vi "CS-4 Status.vi"(0 "VISA session":refnum<visa-resource-name>, 11 "error in (no error)":errorcluster) -> (1 "Magnet Current":string=" +000.000 A                ", 2 "Magnet Voltage":string=" +0.00 V                ", 3 "Output Current":string=" +000.000 A                ", 4 "dup VISA session":refnum<visa-resource-name>, 6 "Output Voltage":string=" +0.00 V                ", 8 "Sweep Mode":string="PAUSED", 9 "sweep states":T1, 10 "Auto Mode":bool=TRUE, 12 "Off Line":bool, 13 "Power Loss":bool, 14 "Quench":bool, 15 "error out":errorcluster)   [LabVIEW 2016]
doc: "CS-4 Status.vi uses the CS-4 driver VI's to monitor the present sensor reading and optionally return status information. If the STB Request option is set TRUE then flags are set to indicate if a quench has been detected or wall power has failed. Off Line is set TRUE if the CS-4 has been placed in Menu or Local modes. The CS-4 will not respond to control commands when off line.\n\nA VISA channel must be opened using CS-4 Initialize.vi before this VI is invoked."
panel:
  out "Cryologo":bool
  # "Model CS-4"
  # "CRYOMAGNETICS, INC."
  # "Magnet Power Supply Status"
  # "Operational Mode"
  # "Sweep Mode"
  # "Flags"
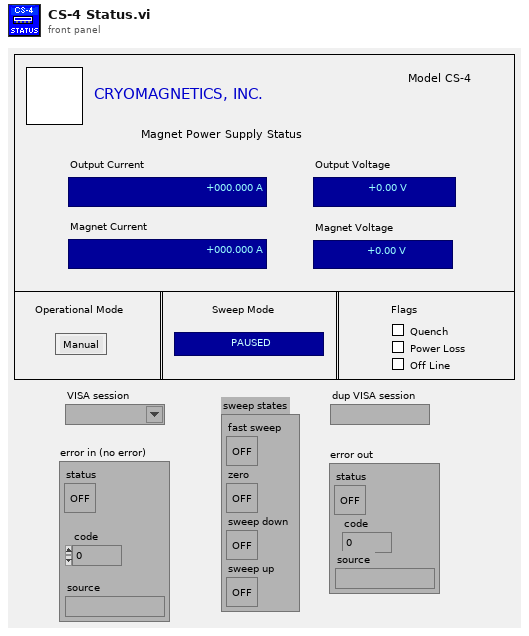
[diagram p1: front panel]
types:
  T1 = cluster{"fast sweep":bool, "zero":bool, "sweep down":bool, "sweep up":bool}
  T2 = cluster{"zero":bool, "sweep up":bool, "sweep down":bool, "fast sweep":bool}
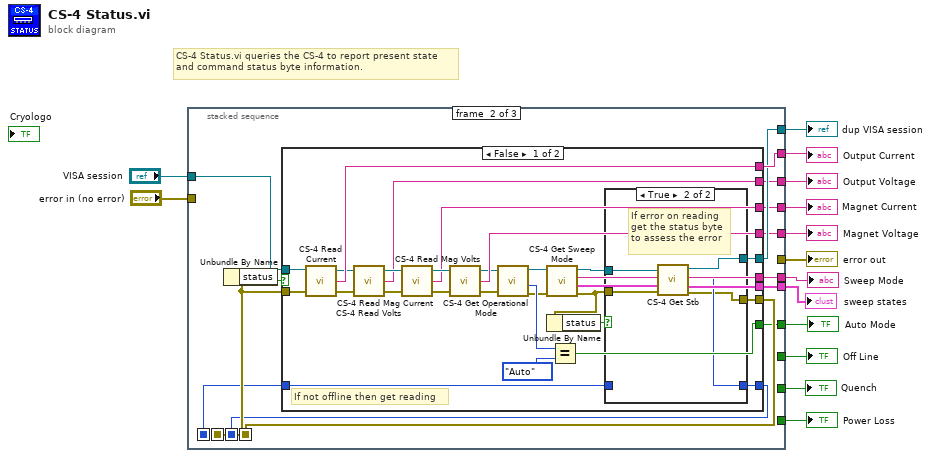
[diagram p0: block diagram]
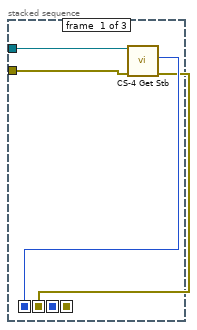
[diagram p2: hidden frame]
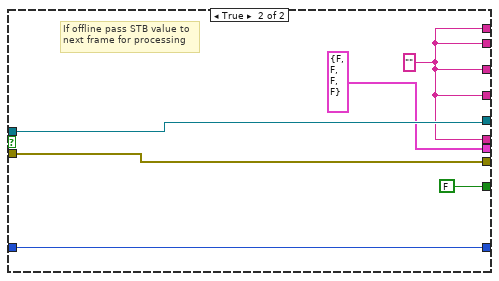
[diagram p4: hidden frame]
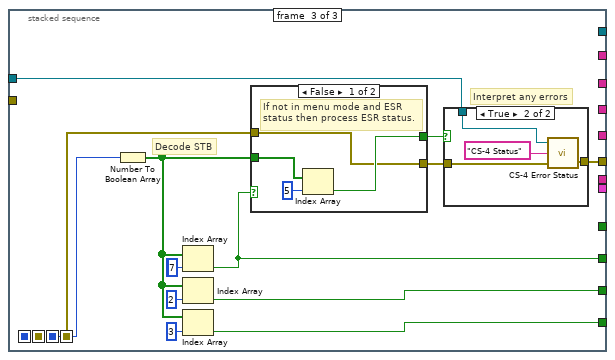
[diagram p5: hidden frame]
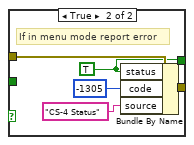
[diagram p6: hidden frame]
diagram:
  # "CS-4 Status.vi queries the CS-4 to report present state \nand command status byte information."
  n1 = stacked-sequence "Sequence" {
    seq-local: [w15 _ _] -> [_ w31 _]
    seq-local: [w17 _ _] -> [_ w27 _]
    seq-local: [_ w26 _] -> [_ _ w75]
    seq-local: [_ w25 _] -> [_ _ w76]
    tunnel: "VISA session" -> [w16 w30 w77]
    tunnel: "error in (no error)" -> [w18 _ _]
    tunnel: [_ _ w87] -> w13
    tunnel: [_ _ w78] -> w12
    tunnel: [_ w29 _] -> w9
    tunnel: [_ w28 _] -> w14
    tunnel: [_ _ w80] -> w8
    tunnel: [_ _ w79] -> w7
    tunnel: [_ w24 _] -> w6
    tunnel: [_ w23 _] -> w5
    tunnel: [_ w22 _] -> w4
    tunnel: [_ w21 _] -> w1
    tunnel: [_ w20 _] -> w3
    tunnel: [_ w19 _] -> w2
    frame #0 {
      n2 = call "CS-4 Get Stb.vi"("error in (no error)"=w18, "VISA session"=w16) -> ("error out"=w15:errorcluster, "stb"=w17:i32)  [unwired: 2 in, 2 out]
    }
    frame #1 {
      n3 = Unbundle By Name(w31) -> ("status"=w32:bool)
      n4 = case shown="False" w32 {
        tunnel: w31 -> [w60 w74]
        tunnel: w30 -> [w59 w73]
        tunnel: [w56 w74] -> w25
        tunnel: [w58 w70] -> w29
        tunnel: [w55 w73] -> w28
        tunnel: [w54 w72] -> w26
        tunnel: w27 -> [w53 w72]
        tunnel: [w46 w70] -> w24
        tunnel: [w45 w70] -> w23
        tunnel: [w44 w70] -> w22
        tunnel: [w35 T1 {"fast sweep"=FALSE, "zero"=FALSE, "sweep down"=FALSE, "sweep up"=FALSE} ("sweep mode")] -> w21
        tunnel: [w36 FALSE] -> w20
        tunnel: [w33 w70] -> w19
        frame False {
          # "If not offline then get reading"
          n5 = call "CS-4 Read Current.vi"("error in (no error)"=w60, "VISA session"=w59) -> ("error out"=w52:errorcluster, "response out"=w58:string, "dup VISA session"=w49:refnum<visa-resource-name>)  [unwired: 1 in]
          n6 = call "CS-4 Read Volts.vi"("error in (no error)"=w52, "VISA session"=w49) -> ("error out"=w51:errorcluster, "response out"=w46:string, "dup VISA session"=w48:refnum<visa-resource-name>)  [unwired: 1 in]
          n7 = call "CS-4 Read Mag Current.vi"("error in (no error)"=w51, "VISA session"=w48) -> ("error out"=w50:errorcluster, "response out"=w45:string, "dup VISA session"=w47:refnum<visa-resource-name>)  [unwired: 1 in]
          n8 = call "CS-4 Read Mag Volts.vi"("error in (no error)"=w50, "VISA session"=w47) -> ("error out"=w43:errorcluster, "response out"=w44:string, "dup VISA session"=w41:refnum<visa-resource-name>)  [unwired: 1 in]
          n9 = call "CS-4 Get Operational Mode.vi"("VISA session"=w41, "error in (no error)"=w43) -> ("dup VISA session"=w40:refnum<visa-resource-name>, "Mode"=w37:enum16{"Manual", "Auto"}, "error out"=w34:errorcluster)  [unwired: 1 in, 1 out]
          n10 = call "CS-4 Get Sweep Mode.vi"("error in (no error)"=w34, "VISA session"=w40) -> ("error out"=w42:errorcluster, "sweep mode"=w35:T2, "response out"=w33:string, "dup VISA session"=w39:refnum<visa-resource-name>)  [unwired: 2 in]
          n11 = Unbundle By Name(w42) -> ("status"=w57:bool)
          n12 = Equal?(x=w37, y=enum16{"Manual", "Auto"}."Auto" ("Mode")) -> (x = y?=w36:bool)
          n13 = case shown="True" w57 {
            tunnel: w42 -> [w62 w67]
            tunnel: w39 -> [w61 w68]
            tunnel: [w63 w65] -> w54
            tunnel: [w62 w64] -> w56
            tunnel: [w61 w66] -> w55
            tunnel: w53 -> [w63 _]
            frame False {
              # "If no error on reading then \npass STB to next frame \nto update device flags"
            }
            frame True {
              # "If error on reading\nget the status byte \nto assess the error"
              n14 = call "CS-4 Get Stb.vi"("error in (no error)"=w67, "VISA session"=w68) -> ("error out"=w64:errorcluster, "stb"=w65:i32, "dup VISA session"=w66:refnum<visa-resource-name>)  [unwired: 2 in, 1 out]
            }
          }
        }
        frame True {
          w70 = "" ("response out")
          # "If offline pass STB value to\nnext frame for processing"
        }
      }
    }
    frame #2 {
      (unwired) 7
      # "Decode STB"
      # "Interpret any errors"
      n15 = Number To Boolean Array(number=w75) -> (Boolean array=w83:bool[])
      n16 = Index Array(array=w83, index=7) -> (element=w78:bool)
      n17 = Index Array(array=w83, index=2) -> (element=w80:bool)
      n18 = Index Array(array=w83, index=3) -> (element=w79:bool)
      n19 = case "Device Offline (in MENU mode)" shown="False" w78 {
        tunnel: [w88 w95] -> w85
        tunnel: w76 -> [w88 w96]
        tunnel: w83 -> [w90 _]
        tunnel: [w89 w92] -> w86
        frame False {
          # "If not in menu mode and ESR\nstatus then process ESR status."
          # "not in Menu mode"
          n20 = Index Array(array=w90, index=5) -> (element=w89:bool)
        }
        frame True {
          w92 = TRUE ("status")
          # "If in menu mode report error"
          # "in Menu mode"
          n21 = Bundle By Name(cluster=w96, "status"=w92, "code"=-1305, "source"="CS-4 Status") -> (w95:errorcluster)
        }
      }
      n22 = case shown="True" w86 {
        tunnel: w77 -> [_ w98]
        tunnel: [w97 w101] -> w87
        tunnel: w85 -> [w97 w99]
        frame False {
        }
        frame True {
          n23 = call "CS-4 Error Status.vi"("error in (no error)"=w99, "VI name"="CS-4 Status", "VISA session"=w98) -> ("error out"=w101:errorcluster)  [unwired: 1 out]
        }
      }
    }
  }
  "Output Current" <- w9
  "error out" <- w13
  "dup VISA session" <- w14
  "Power Loss" <- w7
  "Off Line" <- w12
  "Quench" <- w8
  "Auto Mode" <- w3
  "Sweep Mode" <- w2
  "Magnet Voltage" <- w4
  "Output Voltage" <- w6
  "Magnet Current" <- w5
  "sweep states" <- w1
